vi "ExportConfigurationToFile.vi"(8 "error in (no error)":errorcluster, 11 "Node Ptr":u64 format="%.0x") -> (0 "error out":errorcluster)   [LabVIEW 2025, in "Protection and Counter Addon System Explorer.lvlib"]
uses:
  Protection and Counter Addon System Explorer.lvlib
  <vilib>/NI/NI VeriStand Custom Device Import and Export Tool/ImportExport.lvlib
panel:
  in  "Tag":string
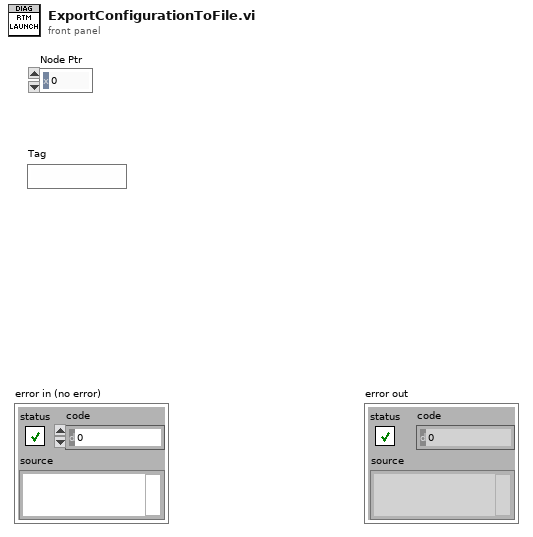
[diagram p1: front panel]
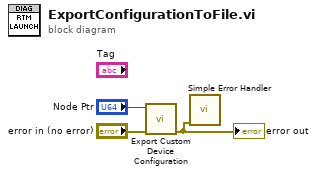
[diagram p0: block diagram]
diagram:
  n1 = call <vilib>:"Export Custom Device Configuration.vi"("error in (no error)"="error in (no error)", "ID"="Node Ptr") -> ("error out"=w1:errorcluster)  [unwired: 8 in, 1 out]
  "error out" <- w1
  n2 = call <vilib>:"Simple Error Handler.vi"("error in (no error)"=w1) -> ()  [unwired: 4 in, 5 out]
